vi "Data file name compatibility manager.vi"(7 "ROI file format version":i32, 9 "ROI number":i32, 10 "Channel A?":bool, 11 "ROI ID string":string) -> (3 "File name":string)   [LabVIEW 2020]
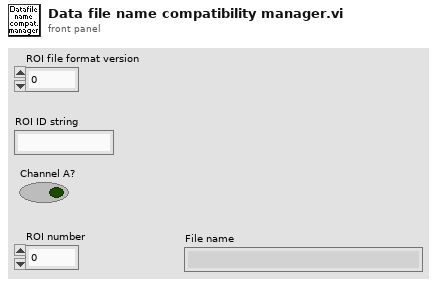
[diagram p1: front panel]
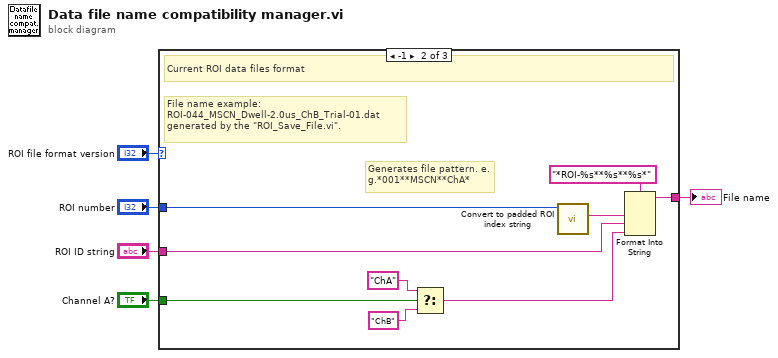
[diagram p0: block diagram]
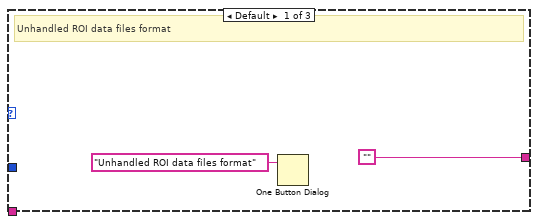
[diagram p2: hidden frame]
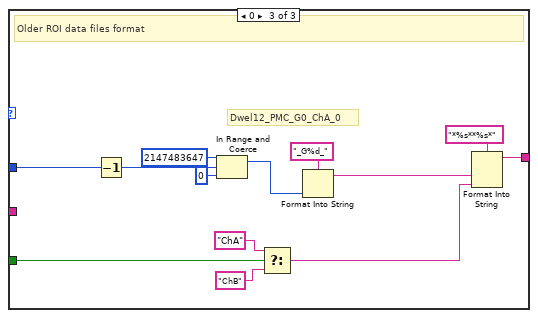
[diagram p3: hidden frame]
diagram:
  n1 = case shown="-1" "ROI file format version" {
    tunnel: "Channel A?" -> [_ w16 w29]
    tunnel: "ROI number" -> [_ w12 w22]
    tunnel: "ROI ID string" -> [_ w11 _]
    tunnel: ["" w10 w25] -> w2
    frame Default {
      # "Unhandled ROI data files format"
      n2 = One Button Dialog(message="Unhandled ROI data files format") -> ()  [unwired: 1 in, 1 out]
    }
    frame -1 {
      # "File name example:\nROI-044_MSCN_Dwell-2.0us_ChB_Trial-01.dat\ngenerated by the \"ROI_Save_File.vi\"."
      # "Generates file pattern. e.g.*001**MSCN**ChA*"
      # "Current ROI data files format"
      n3 = Select(t="ChA" ("string"), s=w16, f="ChB" ("string")) -> (s? t:f=w14:string)
      n4 = call "Convert to padded ROI index string.vi"("ROI number"=w12) -> ("ROI index string padded with zeroes"=w9:string)  [unwired: 10 in]
      n5 = Format Into String(format string="*ROI-%s**%s**%s*" ("pattern"), w9, w11, w14) -> (resulting string=w10:string)  [unwired: 2 in, 1 out]
    }
    frame 0 {
      # "Dwel12_PMC_G0_ChA_0"
      # "Older ROI data files format"
      n6 = Decrement(x=w22) -> (x-1=w20:i32)
      n7 = In Range and Coerce(upper limit=2147483647, x=w20, lower limit=0) -> (coerced(x)=w19:i32)  [unwired: 1 out]
      n8 = Select(t="ChA" ("string"), s=w29, f="ChB" ("string")) -> (s? t:f=w27:string)
      n9 = Format Into String(format string="_G%d_", w19) -> (resulting string=w21:string)  [unwired: 2 in, 1 out]
      n10 = Format Into String(format string="*%s**%s*" ("pattern"), w21, w27) -> (resulting string=w25:string)  [unwired: 2 in, 1 out]
    }
  }
  "File name" <- w2
